vi "TBA_NET_Enable Set.vi"(8 "error in (no error)":errorcluster caption="错误输入（无错误）", 10 "Item[]":T1[](array[typedef]) {"DisplayStyle" items=["None", "Text", "Image", "ImageAndText"]}, 11 "ToolStrip 输入":refnum<class "ToolStrip.lvclass"> caption="Toolbar Ref") -> (0 "error out":errorcluster caption="错误输出", 3 "ToolStrip 输出":refnum<class "ToolStrip.lvclass"> caption="Toolbar Ref Out")   [LabVIEW 2016, in "ToolStrip.lvclass"]
uses:
  Pravite/ToolStrip.lvclass
  TBA_NET_Item.ctl
  Pravite/ToolStrip.lvclass/ToolStrip.ctl
  System.Windows.Forms
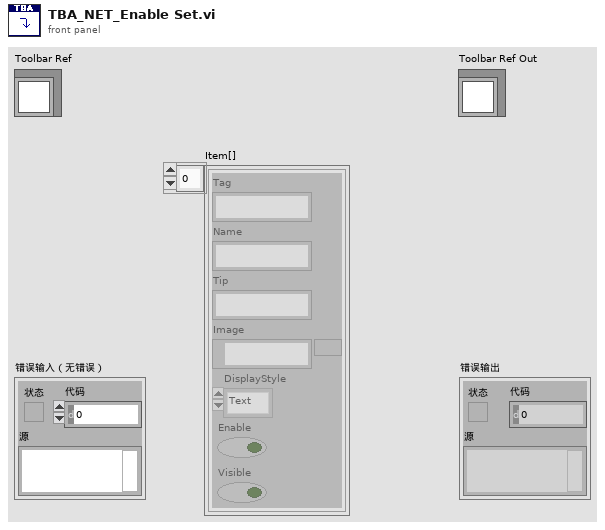
[diagram p1: front panel]
types:
  T1 = typedef "TBA_NET_Item.ctl" = cluster{"Tag":string, "Name":string, "Tip":string, "Image":path, "DisplayStyle":i32, "Enable":bool, "Visible":bool}
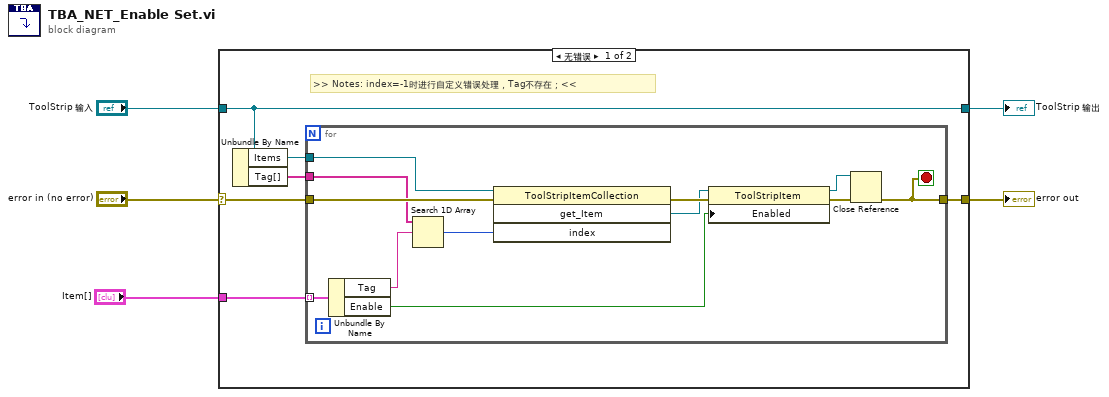
[diagram p0: block diagram]
diagram:
  n1 = case shown="无错误" "error in (no error)" {
    selector: "error in (no error)" -> [w9 w25]
    tunnel: [w8 w25] -> w4
    tunnel: [w11 w24] -> w2
    tunnel: "ToolStrip 输入" -> [w11 w24]
    tunnel: "Item[]" -> [w7 _]
    frame No Error {
      # ">> Notes: index=-1时进行自定义错误处理，Tag不存在；<<"
      n2 = Unbundle By Name(w11) -> ("Items"=w10:refnum<k24>, "Tag[]"=w6:string[])
      n3 = for {
        tunnel: w10 -> [w23]
        tunnel: w9 -> [w22]
        tunnel: [w17] -> w8
        tunnel: w7 -> [w21] mode=indexing
        tunnel: w6 -> [w14]
        stop <- w17 stop-if-true
        n4 = Unbundle By Name(w21) -> ("Tag"=w13:string, "Enable"=w19:bool)
        n5 = Search 1D Array(1D array=w14, element=w13) -> (index of element=w12:i32)  [unwired: 1 in]
        n6 = invoke class="ToolStripItemCollection" method="get_Item"(reference=w23, error in=w22, "index"=w12) -> (error out=w20:errorcluster, "get_Item"=w16:refnum<k24>)  [unwired: 1 in, 2 out]
        n7 = property class="ToolStripItem"(reference=w16, error in=w20, "Enabled"=w19) -> (reference out=w15:refnum<k24>, error out=w18:errorcluster)
        n8 = Close Reference(reference=w15, error in (no error)=w18) -> (error out=w17:errorcluster)
      }
    }
    frame Error {
    }
  }
  "error out" <- w4
  "ToolStrip 输出" <- w2
